vi "niScope Setup Virtual Channels.vi"(4 "samples count":i64=50000 min=1, 6 "fs [Hz]":dbl=50000.0, 7 "trigger setup (Immediate)":T1={"coupling"=1, "level [V]"=0.0, "slope"=0, "mode"=enum."Immediate"} {"level [V]" format="%.2f"; "coupling" items=["AC"=0, "DC"=1, "HF Reject"=3, "LF Reject"=4, "AC Plus HF Reject"=1001]}, 8 "error in":errorcluster, 10 "voltage ranges [Vpk] (empty: use global default)":dbl[](array[numeric]), 11 "niScope in":T4={"channel cfg"=[], "sessions"=[], "multi cards"=FALSE, "channels"=0, "type"=enum."n/a", "memory [B/chn]"=0, "ext. clock [Hz]"=0.0, "samples count"=0, "use streaming"=FALSE, "proc setup"={"packet size [smpl]"=0, "current timeout [s]"=0.0, "blk2blk timeout [s]"=0.0, "event time"=timestamp(0 s since 1904-01-01), "temp sampl T [s]"=0.0, "data queue"=refnum, "stop notifier"=refnum, "proc ref"=refnum}, "sample width [B]"=0, "ranges [V]"=[], "trigger setup"={"coupling"=1, "level [V]"=0.0, "slope"=0, "mode"=enum."Immediate"}, "fs [Hz]"=0.0, "bitres [bit]"=0, "clock source"=enum."VAL_NO_SOURCE"} {"trigger setup"."level [V]" format="%.2f"; "trigger setup"."coupling" items=["AC"=0, "DC"=1, "HF Reject"=3, "LF Reject"=4, "AC Plus HF Reject"=1001]; "channel cfg"."Range [Vpk]" min=0.0; "channel cfg"."Channel" min=0}) -> (0 "error out":errorcluster, 3 "niScope out":T4={"channel cfg"=[], "sessions"=[], "multi cards"=FALSE, "channels"=0, "type"=enum."n/a", "memory [B/chn]"=0, "ext. clock [Hz]"=0.0, "samples count"=0, "use streaming"=FALSE, "proc setup"={"packet size [smpl]"=0, "current timeout [s]"=0.0, "blk2blk timeout [s]"=0.0, "event time"=timestamp(0 s since 1904-01-01), "temp sampl T [s]"=0.0, "data queue"=refnum, "stop notifier"=refnum, "proc ref"=refnum}, "sample width [B]"=0, "ranges [V]"=[], "trigger setup"={"coupling"=1, "level [V]"=0.0, "slope"=0, "mode"=enum."Immediate"}, "fs [Hz]"=0.0, "bitres [bit]"=0, "clock source"=enum."VAL_NO_SOURCE"} {"trigger setup"."level [V]" format="%.2f"; "trigger setup"."coupling" items=["AC"=0, "DC"=1, "HF Reject"=3, "LF Reject"=4, "AC Plus HF Reject"=1001]; "channel cfg"."Range [Vpk]" min=0.0; "channel cfg"."Channel" min=0})   [LabVIEW 2020, in "niScope Virtual Digitizer.lvlib"]
doc: "Configures all virtual channels of the digitizer. Uses global and channel settings from the input session. If vector of voltage ranges in assigned to the function it will override default channel setting from the session. If it is empty, the defaults in the session will be used. Sampling rate and samples count to capture are set by additional inputs. Trigger can be set to other than immediate mode only for single shot mode (for streaming mode it is not yet supported). The VI prepares the cards for acquiring the data. It also implements synchronization via ni-Tclk in case multiple cards are used together. Call this at least once before doing first acquisition. It is not necessary to call this again when multiple acquisitions are performed repetedely with identical settings."
uses:
  niScope Virtual Digitizer.lvlib
  niScope Session.ctl
  niScope Virtual Channel Config.ctl
  niScope Virtual Channel Mode.ctl
  niScope Virtual Channel Input Z.ctl
  niScope Virtual Channel Coupling.ctl
  niScope Type.ctl
  niScope Digitizing Process Options.ctl
  niScope Data Packet.ctl
  niScope Trigger Setup.ctl
  <instrlib>/niScope/Controls/niScope trigger coupling.ctl
  <instrlib>/niScope/Controls/niScope trigger slope.ctl
  niScope Reference Clock.ctl
  <instrlib>/niScope/Controls/niScope vertical coupling.ctl
  <instrlib>/niScope/Controls/niScope trigger source.ctl
  <vilib>/Utility/error.llb/Error Cluster From Error Code.vi
  <instrlib>/niScope/Configure/Trigger/niScope Configure Trigger Edge.vi
  <instrlib>/niScope/Configure/Trigger/niScope Configure Trigger Immediate.vi
  <instrlib>/niScope/Configure/Trigger/niScope Configure Trigger Software.vi
  <vilib>/ErrorRing/Error Ring.xnode
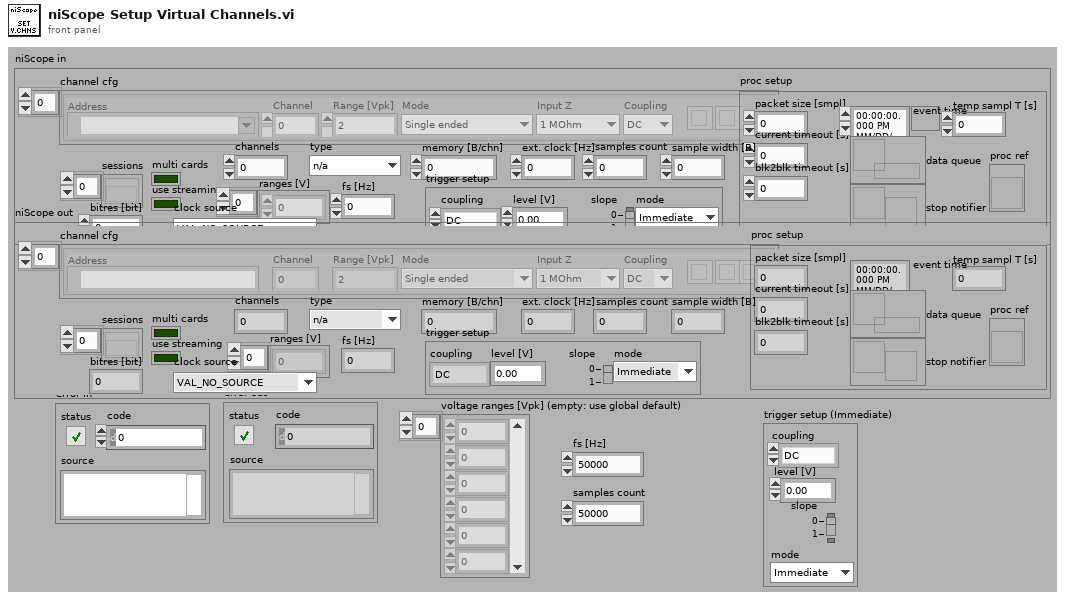
[diagram p1: front panel]
types:
  T1 = typedef "niScope Virtual Digitizer.lvlib/niScope Trigger Setup.ctl" = cluster{"coupling":T2, "level [V]":dbl, "slope":T3, "mode":enum16{"Immediate", "External", "Level"}}
  T2 = typedef "niScope trigger coupling.ctl" = u16
  T3 = typedef "niScope trigger slope.ctl" = i32
  T4 = typedef "niScope Virtual Digitizer.lvlib/niScope Session.ctl" = cluster{"channel cfg":T5[], "sessions":refnum<k20>[], "multi cards":bool, "channels":i32, "type":T9, "memory [B/chn]":i32, "ext. clock [Hz]":dbl, "samples count":i64, "use streaming":bool, "proc setup":T10, "sample width [B]":i32, "ranges [V]":dbl[], "trigger setup":T1, "fs [Hz]":dbl, "bitres [bit]":i32, "clock source":T11}
  T5 = typedef "niScope Virtual Digitizer.lvlib/niScope Virtual Channel Config.ctl" = cluster{"Address":refnum<k15>, "Channel":i32, "Mode":T6, "Input Z":T7, "Coupling":T8, "Range [Vpk]":dbl, "btn clr":bool, "btn up":bool, "btn down":bool}
  T6 = typedef "niScope Virtual Digitizer.lvlib/niScope Virtual Channel Mode.ctl" = enum16{"Single ended", "Unbal. differential", "Differential"}
  T7 = typedef "niScope Virtual Digitizer.lvlib/niScope Virtual Channel Input Z.ctl" = enum16{"1 MOhm", "50 Ohm"}
  T8 = typedef "niScope Virtual Digitizer.lvlib/niScope Virtual Channel Coupling.ctl" = enum16{"AC", "DC", "GND"}
  T9 = typedef "niScope Virtual Digitizer.lvlib/niScope Type.ctl" = enum16{"n/a", "5922"}
  T10 = typedef "niScope Virtual Digitizer.lvlib/niScope Digitizing Process Options.ctl" = cluster{"packet size [smpl]":i64, "current timeout [s]":dbl, "blk2blk timeout [s]":dbl, "event time":timestamp, "temp sampl T [s]":dbl, "data queue":refnum<queue>, "stop notifier":refnum<notifier>, "proc ref":refnum<vi>}
  T11 = typedef "niScope Virtual Digitizer.lvlib/niScope Reference Clock.ctl" = enum16{"VAL_NO_SOURCE", "VAL_CLK_IN", "VAL_PXI_CLOCK", "VAL_EXTERNAL"}
  T12 = typedef "niScope Virtual Digitizer.lvlib/niScope Physical Cards.ctl" = cluster{"chn lst":i32[], "addr":refnum<k15>, "chn pos":i32[]}
  T13 = typedef "niScope trigger source.ctl" = string
  T14 = typedef "niScope vertical coupling.ctl" = i32
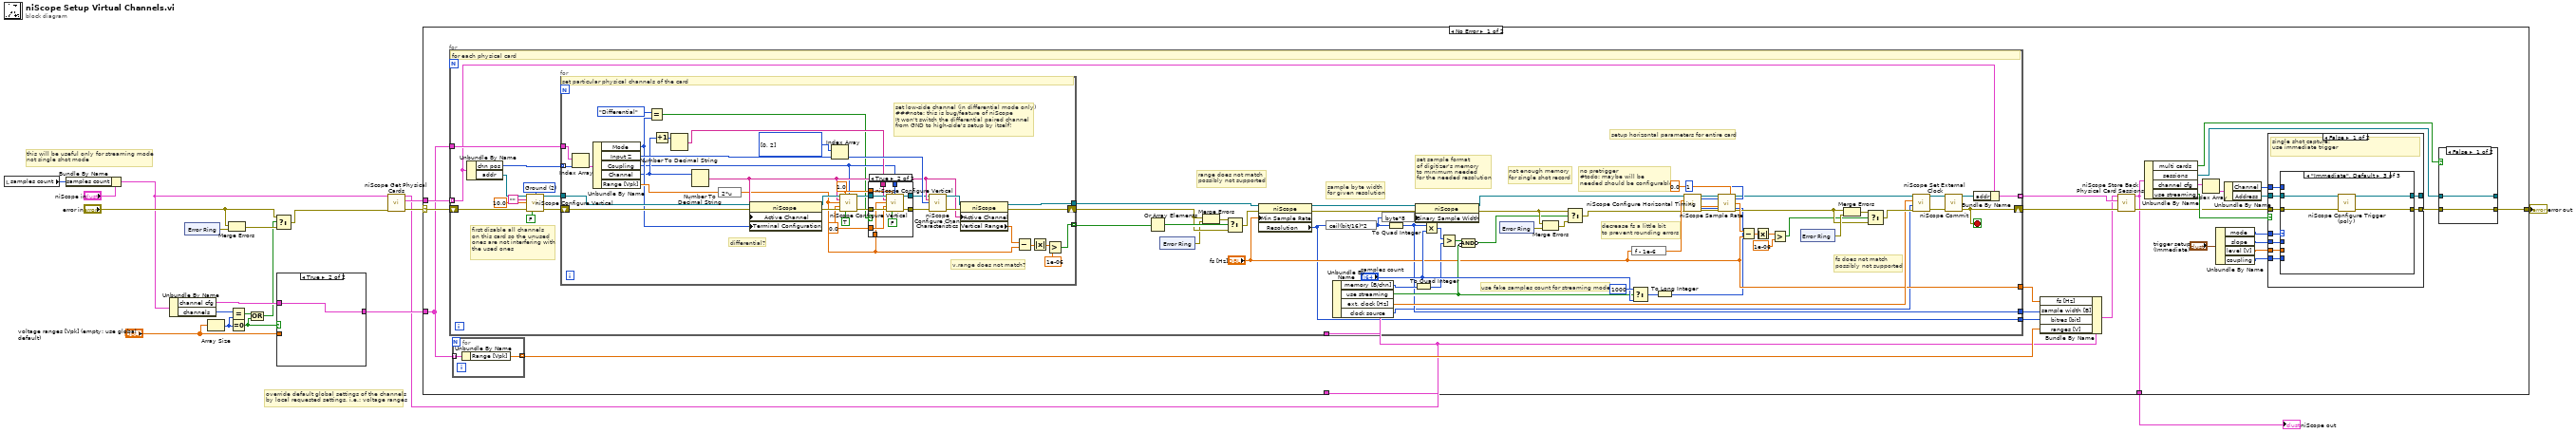
[diagram p0: block diagram]
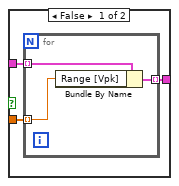
[diagram p2: hidden frame]
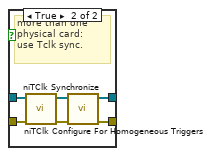
[diagram p3: hidden frame]
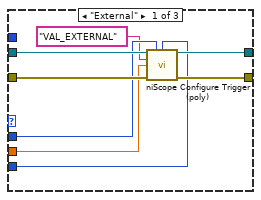
[diagram p4: hidden frame]
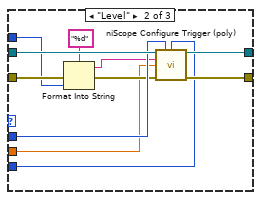
[diagram p5: hidden frame]
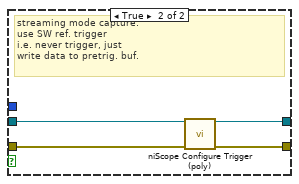
[diagram p6: hidden frame]
diagram:
  # "this will be useful only for streaming mode\nnot single shot mode"
  # "override default global settings of the channels\nby local requested settings, i.e.: voltage ranges"
  n1 = local read "samples count"() -> (w11:i64)
  n2 = Bundle By Name(cluster="niScope in", "samples count"=w11) -> (w9:T4)
  n3 = Unbundle By Name(w9) -> ("channel cfg"=w18:T5[], "channels"=w19:i32)
  n4 = xnode "Error Ring"() -> ("error out"=w15:errorcluster)
  n5 = Array Size(array="voltage ranges [Vpk] (empty: use global default)") -> (size(s)=w6:i32)
  n6 = Merge Errors("error in", w15) -> (w14:errorcluster)
  n7 = Equal?(x=w19, y=w6) -> (x = y?=w7:bool)
  n8 = Equal To 0?(x=w6) -> (x = 0?=w3:bool)
  n9 = Compound Arithmetic op=OR(w7, w3) -> (w5:bool)
  n10 = Select(t="error in", s=w5, f=w14) -> (s? t:f=w2:errorcluster)
  n11 = case shown="True" w3 {
    tunnel: w18 -> [w23 w27]
    tunnel: [w22 w27] -> w17
    tunnel: "voltage ranges [Vpk] (empty: use global default)" -> [w21 _]
    frame False {
      n12 = for {
        tunnel: w23 -> [w26] mode=indexing
        tunnel: w21 -> [w24] mode=indexing
        tunnel: [w25] -> w22 mode=indexing
        n13 = Bundle By Name(cluster=w26, "Range [Vpk]"=w24) -> (w25:T5)
      }
    }
    frame True {
    }
  }
  n14 = call "niScope Get Physical Cards.vi"("error in"=w2, "niScope in"=w9) -> ("error out"=w13:errorcluster, "card list"=w20:T12[], "niScope out"=w8:T4)  [unwired: 7 in]
  n15 = case shown="No Error" w13 {
    selector: w13 -> [w54 w228]
    tunnel: w20 -> [w38 _]
    tunnel: w17 -> [w37 _]
    tunnel: w8 -> [w31 w227]
    tunnel: [w46 w228] -> w10
    tunnel: [w28 w227] -> w1
    frame No Error {
      n16 = for {
        tunnel: w38 -> [w103] mode=indexing
        shift-right: [w135] -> w33
        shift-left: w54 -> [w161]
        tunnel: w37 -> [w155]
        tunnel: w31 -> [w145]
        tunnel: [w109] -> w39
        tunnel: ["fs [Hz]"] -> w35
        tunnel: [w106] -> w34
        tunnel: [w101] -> w30 mode=indexing
        stop <- w135 stop-if-true
        w157 = T14 2 items=["AC", "DC", "Ground"] ("vertical coupling")
        # "set sample format\nof digitizer's memory\nto minimum needed\nfor the needed resolution"
        # "not enough memory\nfor single shot record"
        # "sample byte width\nfor given resolution"
        # "use fake samples count for streaming mode"
        # "fs does not match\npossibly not supported"
        # "setup horizontal parameters for entire card"
        # "range does not match\npossibly not supported"
        # "decrease fs a little bit\nto prevent rounding errors"
        # "no pretrigger\n#todo: maybe will be\nneeded should be configurable"
        # "first disable all channels\non this card so the unused\nones are not interfering with\nthe used ones"
        # "for each physical card"
        n17 = Unbundle By Name(w103) -> ("chn pos"=w163:i32[], "addr"=w160:refnum<k15>)
        n18 = call <instrlib>:"niScope Configure Vertical.vi"("instrument handle"=w160, "vertical coupling"=w157, "channels"="", "vertical range"=10.0, "error in"=w161, "channel enabled"=FALSE) -> ("instrument handle out"=w159:refnum<k15>, "error out"=w162:errorcluster)  [unwired: 8 in]
        n19 = for {
          shift-right: [w199] -> w141
          shift-left: w162 -> [w208]
          tunnel: w163 -> [w214] mode=indexing
          tunnel: w159 -> [w207]
          tunnel: w155 -> [w210]
          tunnel: [w198] -> w126
          tunnel: [w197] -> w144 mode=indexing
          w195 = u32[] [0, 2] items=["1 mega ohm"=0, "50 ohms"=2]
          w181 = 0.0 ("vertical offset")
          w183 = 1.0 ("probe attenuation")
          # "set low-side channel (in differential mode only)\n###note: this is bug/feature of niScope\nIt won't switch the differential paired channel\nfrom GND to high-side's setup by itself!"
          # "v.range does not match?"
          # "differential?"
          # "set particular physical channels of the card"
          n20 = Index Array(array=w210, index=w214) -> (element=w213:T5)
          n21 = Unbundle By Name(w213) -> ("Mode"=w193:T6, "Input Z"=w196:T7, "Coupling"=w182:T8, "Channel"=w191:i32, "Range [Vpk]"=w212:dbl)
          n22 = Equal?(x=niScope_Virtual_Channel_Mode."Differential", y=w193) -> (x = y?=w179:bool)
          n23 = Increment(x=w191) -> (x+1=w189:i32)
          n24 = Number To Decimal String(number=w189) -> (decimal integer string=w184:string)  [unwired: 1 in]
          n25 = Number To Decimal String(number=w191) -> (decimal integer string=w190:string)  [unwired: 1 in]
          n26 = expression code="2*u"(w212) -> (w180:dbl)
          n27 = property class="niScope"(reference=w207, error in=w208, "Active Channel"=w190, "Terminal Configuration"=w193) -> (reference out=w206:refnum<k15>, error out=w209:errorcluster)
          n28 = Index Array(array=w195, index=w196) -> (element=w194:u32)
          n29 = call <instrlib>:"niScope Configure Vertical.vi"("instrument handle"=w206, "probe attenuation"=w183, "vertical coupling"=w182, "channels"=w190, "vertical range"=w180, "vertical offset"=w181, "error in"=w209, "channel enabled"=TRUE) -> ("instrument handle out"=w187:refnum<k15>, "error out"=w188:errorcluster)  [unwired: 6 in]
          n30 = case shown="True" w179 {
            tunnel: w188 -> [w215 w226]
            tunnel: w187 -> [w216 w225]
            tunnel: [w215 w224] -> w186
            tunnel: [w216 w223] -> w185
            tunnel: w184 -> [_ w222]
            tunnel: w183 -> [_ w221]
            tunnel: w182 -> [_ w220]
            tunnel: w181 -> [_ w218]
            tunnel: w180 -> [_ w217]
            frame False {
            }
            frame True {
              n31 = call <instrlib>:"niScope Configure Vertical.vi"("instrument handle"=w225, "probe attenuation"=w221, "vertical coupling"=w220, "channels"=w222, "vertical range"=w217, "vertical offset"=w218, "error in"=w226, "channel enabled"=FALSE) -> ("instrument handle out"=w223:refnum<k15>, "error out"=w224:errorcluster)  [unwired: 6 in]
            }
          }
          n32 = call <instrlib>:"niScope Configure Chan Characteristics.vi"("instrument handle"=w185, "channels"=w190, "input impedance"=w194, "error in"=w186) -> ("instrument handle out"=w204:refnum<k15>, "error out"=w205:errorcluster)  [unwired: 10 in]
          n33 = property class="niScope"(reference=w204, error in=w205, "Active Channel"=w190) -> (reference out=w198:refnum<k15>, error out=w199:errorcluster, "Vertical Range"=w203:dbl)
          n34 = Subtract(x=w203, y=w180) -> (x-y=w202:dbl)
          n35 = Absolute Value(x=w202) -> (abs(x)=w201:dbl)
          n36 = Greater?(x=w201, y=1e-06) -> (0:w197:bool)
        }
        n37 = Or Array Elements(Boolean array=w144) -> (logical OR=w143:bool)
        n38 = xnode "Error Ring"() -> ("error out"=w140:errorcluster)
        n39 = Merge Errors(w141, w140) -> (w142:errorcluster)
        n40 = Select(t=w142, s=w143, f=w141) -> (s? t:f=w127:errorcluster)
        n41 = property class="niScope"(reference=w126, error in=w127, "Min Sample Rate"="fs [Hz]") -> (reference out=w116:refnum<k15>, error out=w117:errorcluster, "Resolution"=w106:i32)
        n42 = expression code="ceil(bit/16)*2"(w106) -> (w111:i32)
        n43 = Unbundle By Name(w145) -> ("memory [B/chn]"=w121:i32, "use streaming"=w119:bool, "ext. clock [Hz]"=w131:dbl, "clock source"=w104:T11)
        n44 = expression code="byte*8"(w111) -> (w115:i32)
        n45 = To Quad Integer(1:w111) -> (0:w109:i64)
        n46 = property class="niScope"(reference=w116, error in=w117, "Binary Sample Width"=w115) -> (reference out=w113:refnum<k15>, error out=w114:errorcluster)
        n47 = To Quad Integer(1:w121) -> (0:w108:i64)
        n48 = Multiply(x=w109, y="samples count") -> (x*y=w122:i64)
        n49 = Greater?(x=w122, y=w108) -> (0:w120:bool)
        n50 = Compound Arithmetic op=AND(w120, invert w119) -> (invert w112:bool)
        n51 = xnode "Error Ring"() -> ("error out"=w124:errorcluster)
        n52 = Merge Errors(w114, w124) -> (w125:errorcluster)
        n53 = Select(t=w114, s=w112, f=w125) -> (s? t:f=w118:errorcluster)
        n54 = expression code="f - 1e-6"("fs [Hz]") -> (w150:dbl)
        n55 = Select(t=i64 1000, s=w119, f="samples count") -> (s? t:f=w129:i64)
        n56 = To Long Integer(number=w129) -> (32bit integer=w107:i32)
        n57 = call <instrlib>:"niScope Configure Horizontal Timing.vi"("instrument handle"=w113, "number of records"=1, "min sample rate"=w150, "reference position"=0.0, "error in"=w118, "min record length"=w107) -> ("instrument handle out"=w149:refnum<k15>, "error out"=w148:errorcluster)  [unwired: 8 in]
        n58 = call <instrlib>:"niScope Sample Rate.vi"("instrument handle"=w149, "error in"=w148) -> ("instrument handle out"=w132:refnum<k15>, "actual sample rate"=w151:dbl, "error out"=w137:errorcluster)  [unwired: 11 in]
        n59 = Subtract(x=w151, y="fs [Hz]") -> (x-y=w152:dbl)
        n60 = Absolute Value(x=w152) -> (abs(x)=w153:dbl)
        n61 = Greater?(x=w153, y=1e-06) -> (0:w136:bool)
        n62 = xnode "Error Ring"() -> ("error out"=w139:errorcluster)
        n63 = Merge Errors(w137, w139) -> (w138:errorcluster)
        n64 = Select(t=w138, s=w136, f=w137) -> (s? t:f=w134:errorcluster)
        n65 = call "niScope Set External Clock.vi"("error in"=w134, "clock source"=w104, "ref. clock rate [Hz] (0: use internal clock)"=w131, "niScope reference in"=w132) -> ("error out"=w133:errorcluster, "reference out"=w105:refnum<k15>)  [unwired: 3 in, 3 out]
        n66 = call <instrlib>:"niScope Commit.vi"("instrument handle"=w105, "error in"=w133) -> ("instrument handle out"=w102:refnum<k15>, "error out"=w135:errorcluster)  [unwired: 12 in]
        n67 = Bundle By Name(cluster=w103, "addr"=w102) -> (w101:T12)
      }
      n68 = for {
        tunnel: w37 -> [w56] mode=indexing
        tunnel: [w55] -> w36 mode=indexing
        n69 = Unbundle By Name(w56) -> ("Range [Vpk]"=w55:dbl)
      }
      n70 = Bundle By Name(cluster=w31, "fs [Hz]"=w35, "sample width [B]"=w39, "bitres [bit]"=w34, "ranges [V]"=w36) -> (w29:T4)
      n71 = call "niScope Store Back Physical Card Sessions.vi"("error in"=w33, "card list"=w30, "niScope in"=w29) -> ("error out"=w32:errorcluster, "niScope out"=w28:T4)  [unwired: 7 in]
      n72 = Unbundle By Name(w28) -> ("multi cards"=w47:bool, "sessions"=w48:refnum<k20>[], "channel cfg"=w53:T5[], "use streaming"=w50:bool)
      n73 = Index Array(array=w53) -> (element=w52:T5)  [unwired: 1 in]
      n74 = Unbundle By Name("trigger setup (Immediate)") -> ("mode"=w44:enum16{"Immediate", "External", "Level"}, "slope"=w43:T3, "level [V]"=w41:dbl, "coupling"=w40:T2)
      n75 = Unbundle By Name(w52) -> ("Channel"=w42:i32, "Address"=w51:refnum<k15>)
      n76 = case shown="False" w50 {
        tunnel: w32 -> [w73 w100]
        tunnel: w51 -> [w72 w99]
        tunnel: [w71 w98] -> w49
        tunnel: [w70 w97] -> _
        tunnel: w44 -> [w69 _]
        tunnel: w43 -> [w68 _]
        tunnel: w42 -> [w67 _]
        tunnel: w41 -> [w66 _]
        tunnel: w40 -> [w65 _]
        frame False {
          # "single shot capture:\nuse immediate trigger"
          n77 = case shown="\"Immediate\", Default" w69 {
            tunnel: w73 -> [w81 w88 w96]
            tunnel: w72 -> [w80 w92 w95]
            tunnel: [w78 w90 w94] -> w71
            tunnel: [w79 w91 w93] -> w70
            tunnel: w68 -> [w77 w89 _]
            tunnel: w67 -> [_ w84 _]
            tunnel: w66 -> [w75 w83 _]
            tunnel: w65 -> [w74 w82 _]
            frame "External" {
              n78 = call-poly <instrlib>:"niScope Configure Trigger (poly).vi"("instrument handle"=w80, "trigger slope"=w77, "trigger coupling"=w74, "trigger source"=T13 "VAL_EXTERNAL", "trigger level"=w75, "error in"=w81) -> ("instrument handle out"=w79:refnum<k15>, "error out"=w78:errorcluster)  [unwired: 8 in]
            }
            frame "Level" {
              n79 = Format Into String(format string="%d", error in=w88, w84) -> (resulting string=w86:string, error out=w87:errorcluster)  [unwired: 1 in]
              n80 = call-poly <instrlib>:"niScope Configure Trigger (poly).vi"("instrument handle"=w92, "trigger slope"=w89, "trigger coupling"=w82, "trigger source"=w86, "trigger level"=w83, "error in"=w87) -> ("instrument handle out"=w91:refnum<k15>, "error out"=w90:errorcluster)  [unwired: 8 in]
            }
            frame "Immediate", Default {
              n81 = call-poly <instrlib>:"niScope Configure Trigger (poly).vi"("instrument handle"=w95, "error in"=w96) -> ("instrument handle out"=w93:refnum<k15>, "error out"=w94:errorcluster)  [unwired: 12 in]
            }
          }
        }
        frame True {
          # "streaming mode capture:\nuse SW ref. trigger\ni.e. never trigger, just\nwrite data to pretrig. buf."
          n82 = call-poly <instrlib>:"niScope Configure Trigger (poly).vi"("instrument handle"=w99, "error in"=w100) -> ("instrument handle out"=w97:refnum<k15>, "error out"=w98:errorcluster)  [unwired: 12 in]
        }
      }
      n83 = case shown="False" w47 {
        tunnel: [w58 w63] -> w46
        tunnel: w49 -> [w58 w62]
        tunnel: w48 -> [w57 w61]
        tunnel: [w57 w59] -> _
        frame False {
        }
        frame True {
          # "more than one\nphysical card:\nuse Tclk sync."
          n84 = call <instrlib>:"niTClk Configure For Homogeneous Triggers.vi"("error in (no error)"=w62, "sessions"=w61) -> ("error out"=w64:errorcluster, "sessions out"=w60:refnum<k20>[])  [unwired: 8 in]
          n85 = call <instrlib>:"niTClk Synchronize.vi"("error in (no error)"=w64, "sessions"=w60) -> ("error out"=w63:errorcluster, "sessions out"=w59:refnum<k20>[])  [unwired: 8 in]
        }
      }
    }
    frame Error {
    }
  }
  "error out" <- w10
  "niScope out" <- w1
